vi "Convert Unit (CDB Array).vi"(4 "Quantity":T1, 5 "error in (no error)":errorcluster, 6 "Target Unit":T2, 7 "Base Unit":T2, 8 "Data":cdb[](array[numeric])) -> (0 "error out":errorcluster, 3 "Converted Data":cdb[](array[numeric]))   [LabVIEW 2023, in "NI_HFNetworkAnalysis.lvlib"]
doc: "Convert an array of double complex values for a specified quantity from a base unit to a new unit."
uses:
  NI_HFNetworkAnalysis.lvlib
  Controls/Unit.ctl
  Controls/Quantity.ctl
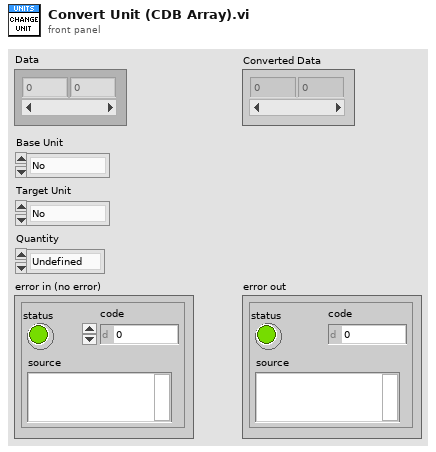
[diagram p1: front panel]
types:
  T1 = typedef "NI_HFNetworkAnalysis.lvlib/Quantity.ctl" = enum16{"Undefined", "V", "I", "A", "B", "P", "Z", "PowerRatio", "Gamma", "Index"}
  T2 = typedef "NI_HFNetworkAnalysis.lvlib/Unit.ctl" = enum16{"No", "s", "Hz", "V", "A", "Ohm", "W", "dB", "dBV", "dBA", "dBm", "percent", "rad", "deg"}
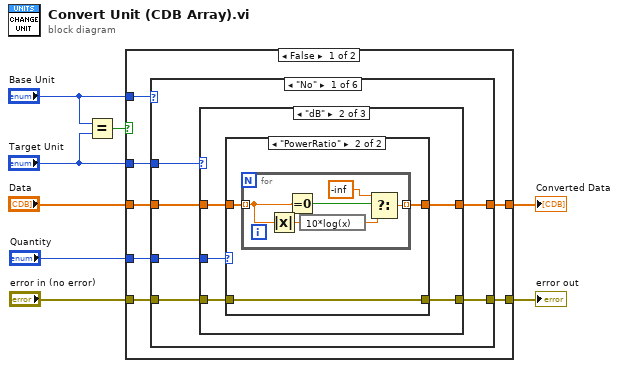
[diagram p0: block diagram]
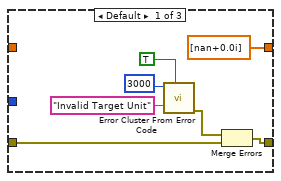
[diagram p2: hidden frame]
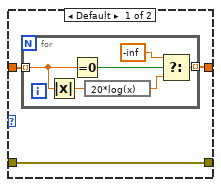
[diagram p3: hidden frame]
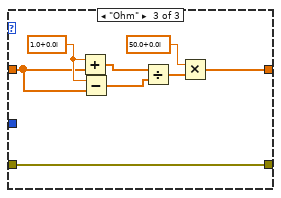
[diagram p4: hidden frame]
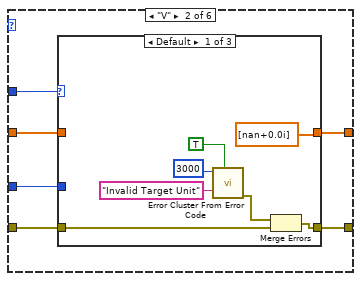
[diagram p5: hidden frame]
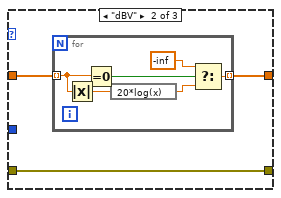
[diagram p6: hidden frame]
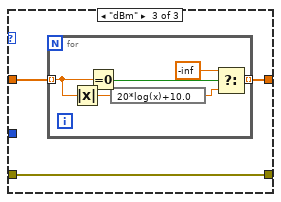
[diagram p7: hidden frame]
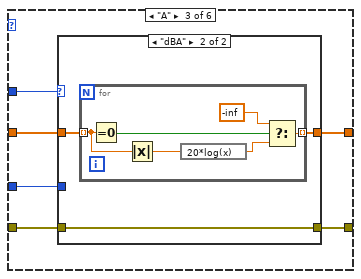
[diagram p8: hidden frame]
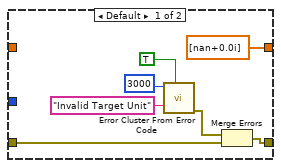
[diagram p9: hidden frame]
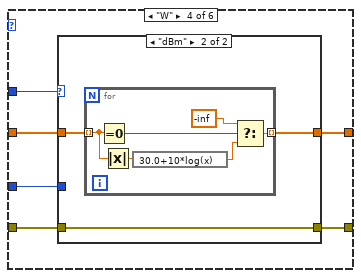
[diagram p10: hidden frame]
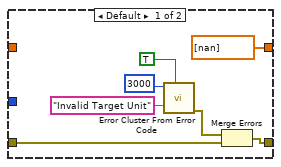
[diagram p11: hidden frame]
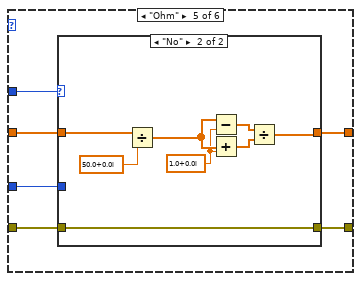
[diagram p12: hidden frame]
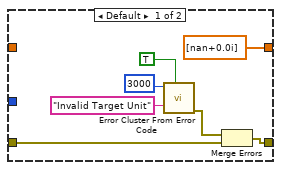
[diagram p13: hidden frame]
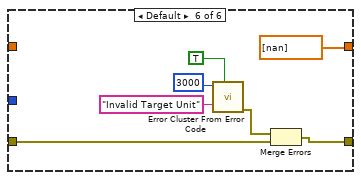
[diagram p14: hidden frame]
diagram:
  n1 = Equal?(x="Base Unit", y="Target Unit") -> (x = y?=w8:bool)
  n2 = case shown="False" w8 {
    tunnel: "Base Unit" -> [w15 _]
    tunnel: [w10 w164] -> w5
    tunnel: "Data" -> [w11 w164]
    tunnel: "Quantity" -> [w14 _]
    tunnel: "error in (no error)" -> [w13 w163]
    tunnel: [w12 w163] -> w2
    tunnel: "Target Unit" -> [w9 _]
    frame False {
      n3 = case shown="\"No\"" w15 {
        tunnel: w14 -> [w21 w65 w96 w118 w140 _]
        tunnel: w13 -> [w20 w64 w95 w117 w139 w162]
        tunnel: [w19 w63 w94 w116 w138 w161] -> w12
        tunnel: w11 -> [w18 w62 w93 w115 w137 _]
        tunnel: [w17 w61 w92 w114 w136 dbl[] [nan] ("Data")] -> w10
        tunnel: w9 -> [w16 w60 w91 w113 w135 _]
        frame "No" {
          n4 = case shown="\"dB\"" w16 {
            tunnel: w21 -> [_ w33 _]
            tunnel: w20 -> [w27 w32 w59]
            tunnel: [w28 w31 w59] -> w19
            tunnel: w18 -> [_ w30 w57]
            tunnel: [cdb[] [nan+0.0i] ("Data") w29 w52] -> w17
            frame Default {
              n5 = call <vilib>:"Error Cluster From Error Code.vi"("show call chain? (False)"=TRUE, "error message (\"\")"="Invalid Target Unit" ("error message (\"\")"), "error code (0)"=3000) -> ("error out"=w26:errorcluster)  [unwired: 6 in]
              n6 = Merge Errors(w26, w27) -> (w28:errorcluster)
            }
            frame "dB" {
              n7 = case shown="\"PowerRatio\"" w33 {
                tunnel: [w36 w45] -> w31
                tunnel: w32 -> [w36 w45]
                tunnel: w30 -> [w34 w44]
                tunnel: [w35 w43] -> w29
                frame Default {
                  n8 = for {
                    tunnel: [w41] -> w35 mode=indexing
                    tunnel: w34 -> [w38] mode=indexing
                    n9 = Absolute Value(x=w38) -> (abs(x)=w42:dbl)
                    n10 = Equal To 0?(x=w38) -> (x = 0?=w39:bool)
                    n11 = expression code="20*log(x)"(w42) -> (w40:dbl)
                    n12 = Select(t=-inf, s=w39, f=w40) -> (s? t:f=w41:dbl)
                  }
                }
                frame "PowerRatio" {
                  n13 = for {
                    tunnel: w44 -> [w50] mode=indexing
                    tunnel: [w49] -> w43 mode=indexing
                    n14 = Absolute Value(x=w50) -> (abs(x)=w51:dbl)
                    n15 = Equal To 0?(x=w50) -> (x = 0?=w47:bool)
                    n16 = expression code="10*log(x)"(w51) -> (w48:dbl)
                    n17 = Select(t=-inf, s=w47, f=w48) -> (s? t:f=w49:dbl)
                  }
                }
              }
            }
            frame "Ohm" {
              w58 = cdb 1.0+0.0i ("x")
              n18 = Add(x=w58, y=w57) -> (x+y=w56:cdb[])
              n19 = Subtract(x=w58, y=w57) -> (x-y=w55:cdb[])
              n20 = Divide(x=w56, y=w55) -> (x/y=w54:cdb[])
              n21 = Multiply(x=cdb 50.0+0.0i, y=w54) -> (x*y=w52:cdb[])
            }
          }
        }
        frame "V" {
          n22 = case shown="Default" w60 {
            tunnel: w65 -> [_ _ _]
            tunnel: w64 -> [w71 w75 w84]
            tunnel: [w72 w75 w84] -> w63
            tunnel: w62 -> [_ w74 w83]
            tunnel: [cdb[] [nan+0.0i] ("Data") w73 w82] -> w61
            frame Default {
              n23 = call <vilib>:"Error Cluster From Error Code.vi"("show call chain? (False)"=TRUE, "error message (\"\")"="Invalid Target Unit" ("error message (\"\")"), "error code (0)"=3000) -> ("error out"=w70:errorcluster)  [unwired: 6 in]
              n24 = Merge Errors(w70, w71) -> (w72:errorcluster)
            }
            frame "dBV" {
              n25 = for {
                tunnel: w74 -> [w80] mode=indexing
                tunnel: [w76] -> w73 mode=indexing
                n26 = Absolute Value(x=w80) -> (abs(x)=w81:dbl)
                n27 = Equal To 0?(x=w80) -> (x = 0?=w78:bool)
                n28 = expression code="20*log(x)"(w81) -> (w79:dbl)
                n29 = Select(t=-inf, s=w78, f=w79) -> (s? t:f=w76:dbl)
              }
            }
            frame "dBm" {
              n30 = for {
                tunnel: w83 -> [w89] mode=indexing
                tunnel: [w87] -> w82 mode=indexing
                n31 = Absolute Value(x=w89) -> (abs(x)=w90:dbl)
                n32 = Equal To 0?(x=w89) -> (x = 0?=w86:bool)
                n33 = expression code="20*log(x)+10.0"(w90) -> (w88:dbl)
                n34 = Select(t=-inf, s=w86, f=w88) -> (s? t:f=w87:dbl)
              }
            }
          }
        }
        frame "A" {
          n35 = case shown="\"dBA\"" w91 {
            tunnel: w96 -> [_ _]
            tunnel: w95 -> [w102 w106]
            tunnel: [w103 w106] -> w94
            tunnel: w93 -> [_ w105]
            tunnel: [cdb[] [nan+0.0i] ("Data") w104] -> w92
            frame Default {
              n36 = call <vilib>:"Error Cluster From Error Code.vi"("show call chain? (False)"=TRUE, "error message (\"\")"="Invalid Target Unit" ("error message (\"\")"), "error code (0)"=3000) -> ("error out"=w101:errorcluster)  [unwired: 6 in]
              n37 = Merge Errors(w101, w102) -> (w103:errorcluster)
            }
            frame "dBA" {
              n38 = for {
                tunnel: w105 -> [w111] mode=indexing
                tunnel: [w108] -> w104 mode=indexing
                n39 = Equal To 0?(x=w111) -> (x = 0?=w109:bool)
                n40 = Absolute Value(x=w111) -> (abs(x)=w112:dbl)
                n41 = expression code="20*log(x)"(w112) -> (w110:dbl)
                n42 = Select(t=-inf, s=w109, f=w110) -> (s? t:f=w108:dbl)
              }
            }
          }
        }
        frame "W" {
          n43 = case shown="\"dBm\"" w113 {
            tunnel: w118 -> [_ _]
            tunnel: w117 -> [w124 w128]
            tunnel: [w125 w128] -> w116
            tunnel: w115 -> [_ w127]
            tunnel: [dbl[] [nan] ("Data") w126] -> w114
            frame Default {
              n44 = call <vilib>:"Error Cluster From Error Code.vi"("show call chain? (False)"=TRUE, "error message (\"\")"="Invalid Target Unit" ("error message (\"\")"), "error code (0)"=3000) -> ("error out"=w123:errorcluster)  [unwired: 6 in]
              n45 = Merge Errors(w123, w124) -> (w125:errorcluster)
            }
            frame "dBm" {
              n46 = for {
                tunnel: w127 -> [w129] mode=indexing
                tunnel: [w132] -> w126 mode=indexing
                n47 = Equal To 0?(x=w129) -> (x = 0?=w134:bool)
                n48 = Absolute Value(x=w129) -> (abs(x)=w130:dbl)
                n49 = expression code="30.0+10*log(x)"(w130) -> (w131:dbl)
                n50 = Select(t=-inf, s=w134, f=w131) -> (s? t:f=w132:dbl)
              }
            }
          }
        }
        frame "Ohm" {
          n51 = case shown="\"No\"" w135 {
            tunnel: w140 -> [_ _]
            tunnel: w139 -> [w146 w155]
            tunnel: [w147 w155] -> w138
            tunnel: w137 -> [_ w154]
            tunnel: [cdb[] [nan+0.0i] ("Data") w149] -> w136
            frame Default {
              n52 = call <vilib>:"Error Cluster From Error Code.vi"("show call chain? (False)"=TRUE, "error message (\"\")"="Invalid Target Unit" ("error message (\"\")"), "error code (0)"=3000) -> ("error out"=w145:errorcluster)  [unwired: 6 in]
              n53 = Merge Errors(w145, w146) -> (w147:errorcluster)
            }
            frame "No" {
              w148 = cdb 1.0+0.0i
              n54 = Divide(x=w154, y=cdb 50.0+0.0i) -> (x/y=w152:cdb[])
              n55 = Subtract(x=w152, y=w148) -> (x-y=w151:cdb[])
              n56 = Add(x=w152, y=w148) -> (x+y=w150:cdb[])
              n57 = Divide(x=w151, y=w150) -> (x/y=w149:cdb[])
            }
          }
        }
        frame Default {
          n58 = call <vilib>:"Error Cluster From Error Code.vi"("show call chain? (False)"=TRUE, "error message (\"\")"="Invalid Target Unit" ("error message (\"\")"), "error code (0)"=3000) -> ("error out"=w160:errorcluster)  [unwired: 6 in]
          n59 = Merge Errors(w160, w162) -> (w161:errorcluster)
        }
      }
    }
    frame True {
    }
  }
  "Converted Data" <- w5
  "error out" <- w2
